vi "Destroy User Events.vi"(8 "error in (no error)":errorcluster, 11 "User Events":T1) -> (0 "error out":errorcluster)   [LabVIEW 2020, in "User Events.lvlib"]
doc: "Destroy the user event, even if there is an incoming error."
uses:
  User Events.lvlib
  controls/User Events ---typedef.ctl
  controls/Wake HL ---argument.ctl
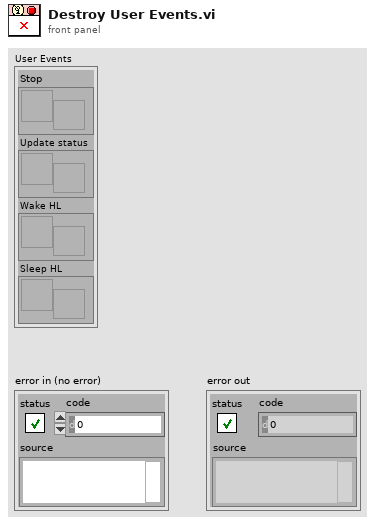
[diagram p1: front panel]
types:
  T1 = typedef "User Events ---typedef.ctl" = cluster{"Stop":refnum<user-event>, "Update status":refnum<user-event>, "Wake HL":refnum<user-event>, "Sleep HL":refnum<user-event>}
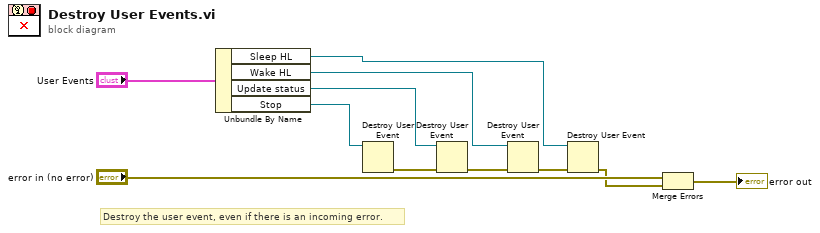
[diagram p0: block diagram]
diagram:
  # "Destroy the user event, even if there is an incoming error."
  n1 = Unbundle By Name("User Events") -> ("Sleep HL"=w2:refnum<user-event>, "Wake HL"=w3:refnum<user-event>, "Update status"=w7:refnum<user-event>, "Stop"=w8:refnum<user-event>)
  n2 = Destroy User Event(user event=w8) -> (error out=w6:errorcluster)  [unwired: 1 in]
  n3 = Destroy User Event(user event=w7, error in=w6) -> (error out=w4:errorcluster)
  n4 = Destroy User Event(user event=w3, error in=w4) -> (error out=w5:errorcluster)
  n5 = Destroy User Event(user event=w2, error in=w5) -> (error out=w1:errorcluster)
  n6 = Merge Errors("error in (no error)", w1) -> (→"error out":errorcluster)
